vi "Limelight Set Stream Mode.vi"(11 "Camra":bool) -> ()   [LabVIEW 2020]
uses:
  <vilib>/Rock Robotics/Network Tables/NT Write Number.vi
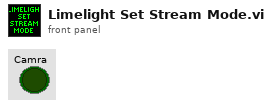
[diagram p1: front panel]
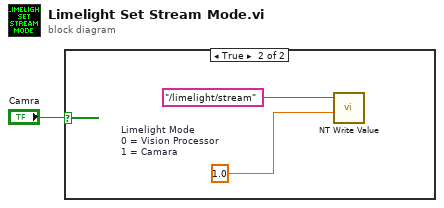
[diagram p0: block diagram]
diagram:
  n1 = case shown="True" "Camra" {
    frame False {
    }
    frame True {
      w2 = 1.0  # Limelight Mode 0 = Vision Processor 1 = Camara
      n2 = call-poly <vilib>:"NT Write Value.vi"("Numeric"=w2, "Name"="/limelight/stream") -> ()  [unwired: 9 in, 1 out]
    }
  }
